vi "Check image quality.vi"(8 "error in (no error)":errorcluster, 11 "Retiga in":refnum<class "Retiga.lvclass">) -> (0 "error out":errorcluster, 2 "QC passed?":bool, 3 "Retiga out":refnum<class "Retiga.lvclass">)   [LabVIEW 2012, in "Retiga.lvclass"]
uses:
  Retiga.lvclass
  Retiga.lvclass/Retiga.ctl
  <vilib>/vision/NI_Vision_Development_Module.lvlib
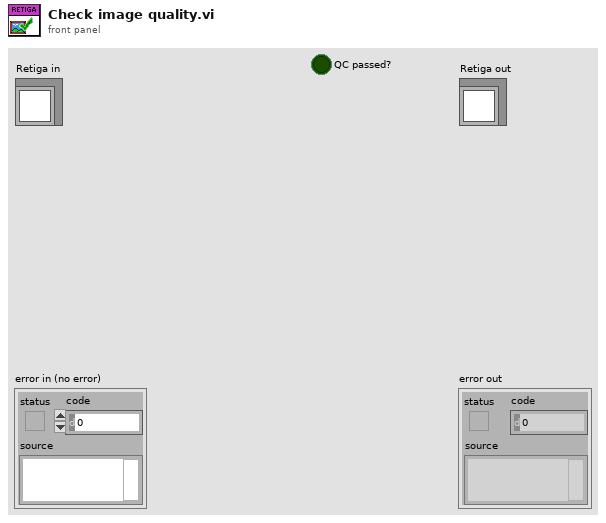
[diagram p1: front panel]
types:
  T1 = typedef "IMAQ Image.ctl" = refnum<image>
  T2 = cluster{"histogram":u32[], "Minimal Value":sgl, "Maximal Value":sgl, "Starting Value":sgl, "Interval Width":sgl, "Mean Value":sgl, "Standard  Variation":sgl, "Area (pixels)":i32}
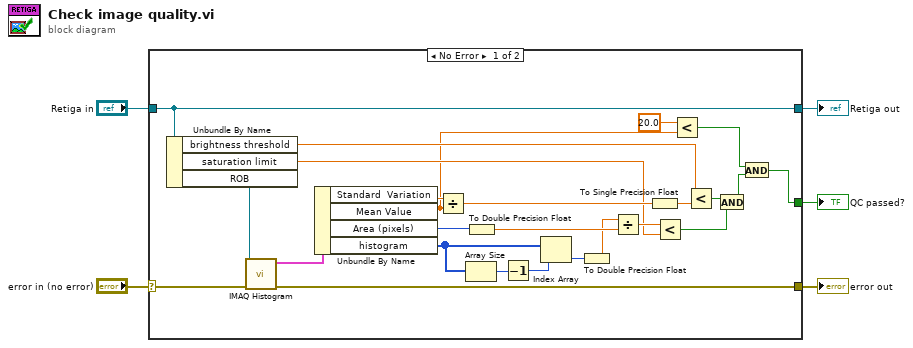
[diagram p0: block diagram]
diagram:
  n1 = case shown="No Error" "error in (no error)" {
    selector: "error in (no error)" -> [w12 w32]
    tunnel: [w11 w32] -> w4
    tunnel: [w16 w31] -> w2
    tunnel: "Retiga in" -> [w16 w31]
    tunnel: [w6 _] -> w1
    frame No Error {
      n2 = Unbundle By Name(w16) -> ("brightness threshold"=w14:sgl, "saturation limit"=w13:dbl, "ROB"=w15:T1)
      n3 = call "IMAQ Histogram"("error in (no error)"=w12, "Image"=w15) -> ("error out"=w11:errorcluster, "Histogram Report"=w29:T2)  [unwired: 8 in]
      n4 = Unbundle By Name(w29) -> ("Standard  Variation"=w28:sgl, "Mean Value"=w10:sgl, "Area (pixels)"=w23:i32, "histogram"=w26:u32[])
      n5 = Divide(x=w28, y=w10) -> (x/y=w27:sgl)
      n6 = Array Size(array=w26) -> (size(s)=w25:i32)
      n7 = To Double Precision Float(number=w23) -> (double precision float=w21:dbl)
      n8 = Decrement(x=w25) -> (x-1=w24:i32)
      n9 = Index Array(array=w26, index=w24) -> (element=w22:u32)
      n10 = To Double Precision Float(number=w22) -> (double precision float=w19:dbl)
      n11 = Divide(x=w19, y=w21) -> (x/y=w20:dbl)
      n12 = To Single Precision Float(number=w27) -> (single precision float=w30:sgl)
      n13 = Less?(x=w20, y=w13) -> (x < y?=w18:bool)
      n14 = Less?(x=sgl 20.0, y=w10) -> (x < y?=w7:bool)
      n15 = Less?(x=w14, y=w30) -> (x < y?=w17:bool)
      n16 = And(x=w17, y=w18) -> (x .and. y?=w8:bool)
      n17 = And(x=w7, y=w8) -> (x .and. y?=w6:bool)
    }
    frame Error {
    }
  }
  "error out" <- w4
  "Retiga out" <- w2
  "QC passed?" <- w1
